vi "Snake Add Score.vi"(8 "error in (no error)":errorcluster, 10 "Amount":u32, 11 "Snake in":refnum<class "Snake.lvclass">) -> (0 "error out":errorcluster, 3 "Snake out":refnum<class "Snake.lvclass">)   [LabVIEW 2020, in "Snake.lvclass"]
uses:
  Snake.lvclass
  Snake.lvclass/Snake.ctl
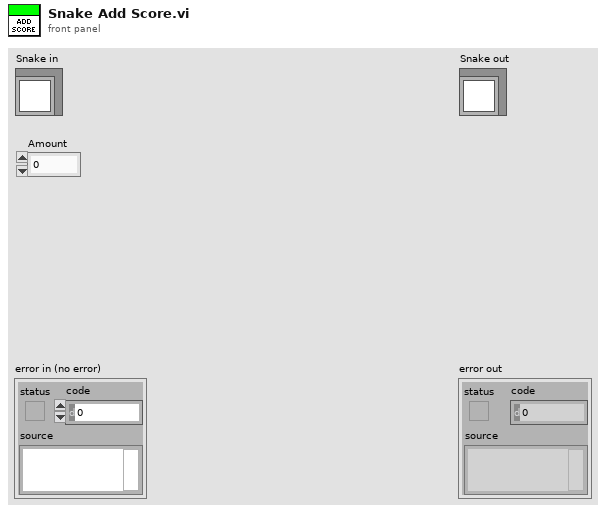
[diagram p1: front panel]
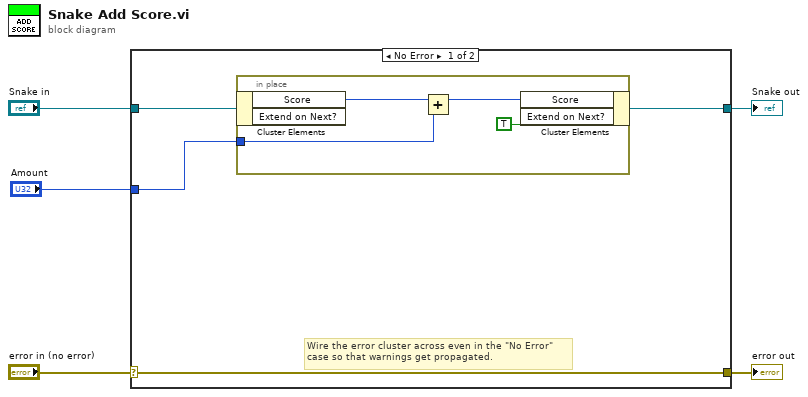
[diagram p0: block diagram]
diagram:
  n1 = case shown="No Error" "error in (no error)" {
    selector: "error in (no error)" -> [w8 w15]
    tunnel: [w8 w15] -> w4
    tunnel: [w7 w14] -> w2
    tunnel: "Snake in" -> [w9 w14]
    tunnel: "Amount" -> [w6 _]
    frame No Error {
      # "Wire the error cluster across even in the \"No Error\"\ncase so that warnings get propagated."
      n2 = in-place {
        in-place-border: w6 -> [w11]
        n3 = in-place-cluster #1(w9) -> ("Score"=w13:u32)  [unwired: 1 out]
        n4 = Add(x=w13, y=w11) -> (x+y=w12:u32)
        n5 = in-place-cluster #1("Score"=w12, "Extend on Next?"=TRUE) -> (w7:refnum<class "Snake.lvclass">)
      }
    }
    frame Error {
    }
  }
  "error out" <- w4
  "Snake out" <- w2
